vi "Allowed root paths.vi"() -> (3 "Allowed root paths":string[](array[string]))   [LabVIEW 2020]
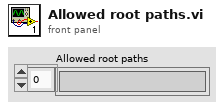
[diagram p1: front panel]
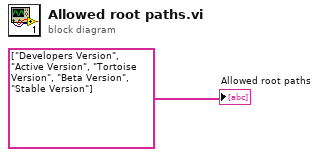
[diagram p0: block diagram]
diagram:
  "Allowed root paths" <- string[] ["Developers Version", "Active Version", "Tortoise Version", "Beta Version", "Stable Version"]
